vi "Initialize.vi"(7 "Channel Name":string="ActualValue.ch%d.AV", 8 "error in":errorcluster, 9 "Number of Channels":u32=1, 10 "Instance Name":string, 11 "Voltage Nominal Value in":refnum<class "Voltage Nominal Value.lvclass">) -> (0 "error out":errorcluster, 2 "Channel":T1[](array[typedef]), 3 "Voltage Nominal Value out":refnum<class "Voltage Nominal Value.lvclass">)   [LabVIEW 2023, in "Voltage Nominal Value.lvclass"]
uses:
  Voltage Nominal Value.lvclass
  Utilities/Channel.ctl
  Parents/Nominal Value/Nominal Value.lvclass
  Utilities/Utilities.lvlib
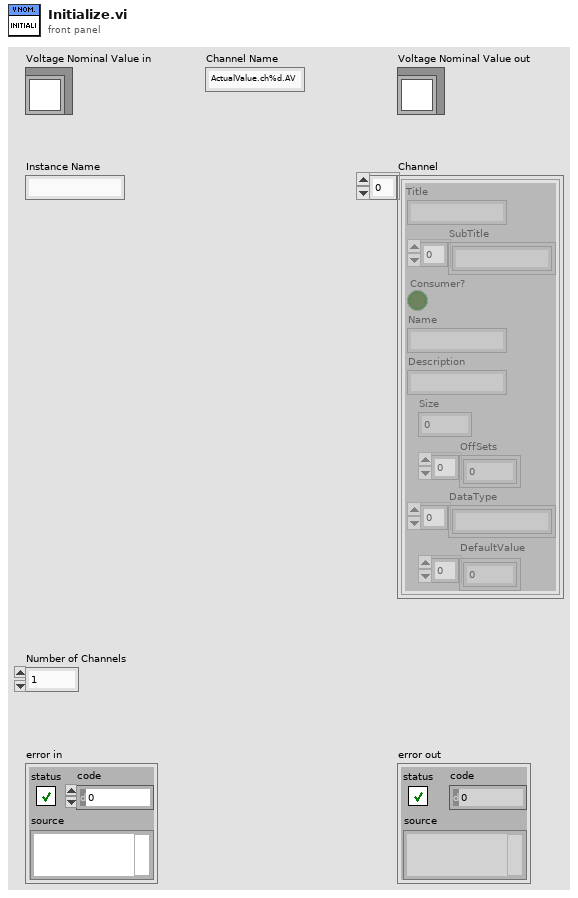
[diagram p1: front panel]
types:
  T1 = typedef "Utilities.lvlib/Channel.ctl" = cluster{"Title":string, "SubTitle":string[], "Consumer?":bool, "Name":string, "Description":string, "Size":i32, "OffSets":i32[], "DataType":string[], "DefaultValue":dbl[]}
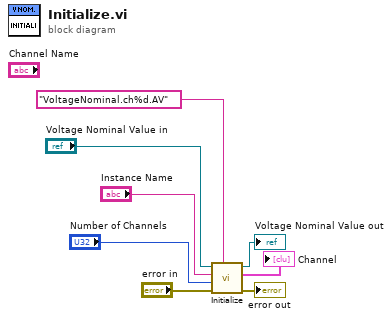
[diagram p0: block diagram]
diagram:
  n1 = call-parent "Initialize.vi"("Channel Name"="VoltageNominal.ch%d.AV" ("ChannelName"), "error in"="error in", "Number of Channels"="Number of Channels", "Instance Name"="Instance Name", "Nominal Value in"="Voltage Nominal Value in") -> ("error out"=→"error out":errorcluster, "Channel"=→"Channel":T1[], "Nominal Value out"=→"Voltage Nominal Value out":refnum<class "Voltage Nominal Value.lvclass">)  [unwired: 4 in]
